vi "Encrypt.vi"(8 "error in (no error)":errorcluster, 10 "input":string, 11 "srp":T1) -> (0 "error out":errorcluster, 1 "IV":u8[](array[numeric]), 2 "output":u8[](array[numeric]), 3 "srp out":T1)   [LabVIEW 2017, in "SRP.lvlib"]
uses:
  <vilib>/addons/InsightCM/SRP/SRP.lvlib
  <vilib>/addons/InsightCM/SRP/controls/DVR_data.ctl
  <vilib>/addons/InsightCM/SRP/controls/data.ctl
  <vilib>/addons/InsightCM/SRP/libraries/win32Urelease/brsrp.dll
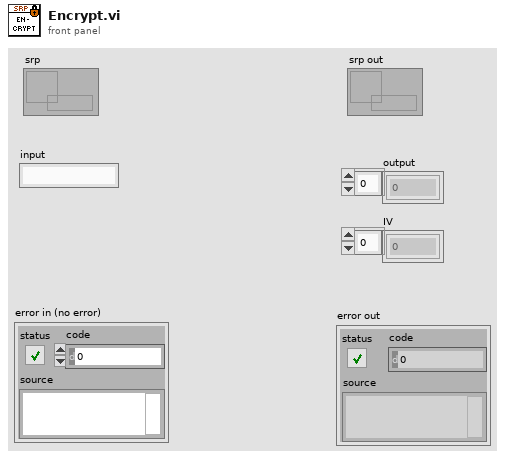
[diagram p1: front panel]
types:
  T1 = typedef "SRP.lvlib/DVR_data.ctl" = refnum<data-value>
  T2 = typedef "SRP.lvlib/data.ctl" = cluster{"SessionKey":u8[], "ClientHash":u8[], "PublicKeyA":u8[], "PrivateKeyA":u8[]}
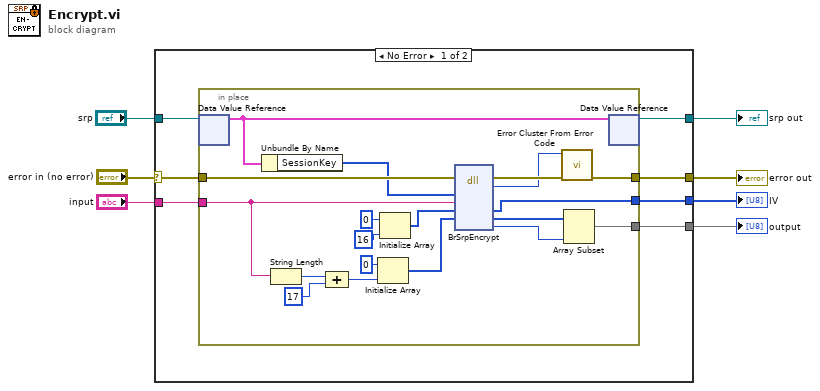
[diagram p0: block diagram]
diagram:
  n1 = case shown="No Error" "error in (no error)" {
    selector: "error in (no error)" -> [w13 w35]
    tunnel: [w14 w35] -> w7
    tunnel: "input" -> [w12 _]
    tunnel: "srp" -> [w11 w34]
    tunnel: [w10 w34] -> w3
    tunnel: [w9 _] -> w2
    tunnel: [w8 _] -> w1
    frame No Error {
      n2 = in-place {
        in-place-border: [w26] -> w14
        in-place-border: w13 -> [w20]
        in-place-border: w12 -> [w19]
        in-place-border: [w16] -> w9
        in-place-border: [w15] -> w8
        n3 = in-place-dvr #1(w11) -> (w17:T2)  [unwired: 1 out]
        n4 = Unbundle By Name(w17) -> ("SessionKey"=w18:u8[])
        n5 = String Length(string=w19) -> (length=w32:i32)
        n6 = Compound Arithmetic op=ADD(w32, 17 ("value")) -> (w28:i32)
        n7 = Initialize Array(u8 0 ("dimension size"), w28) -> (w30:u8[])
        n8 = Initialize Array(u8 0 ("dimension size"), 16 ("dimension size")) -> (w22:u8[])
        n9 = dll-call lib="C:/Program Files (x86)/National Instruments/LabVIEW 2017/vi.lib/addons/InsightCM/SRP/libraries/win32Urelease/brsrp.*" fn="BrSrpEncrypt"(error in=w20, "key"=w18, "input"=w19, "IV"=w22, "output"=w30) -> (error out=w33:errorcluster, "return type"=w25:i32, "IV"=w15:u8[], "output"=w27:u8[], "length"=w24:u32)  [unwired: 5 in, 1 out]
        n10 = call <vilib>:"Error Cluster From Error Code.vi"("error in (no error)"=w33, "error code (0)"=w25) -> ("error out"=w26:errorcluster)  [unwired: 7 in]
        n11 = Array Subset(array=w27, length=w24) -> (w16:u8[])  [unwired: 1 in]
        n12 = in-place-dvr #1(w17) -> (w10:T1)  [unwired: 1 out]
      }
    }
    frame Error {
    }
  }
  "error out" <- w7
  "srp out" <- w3
  "IV" <- w1
  "output" <- w2
